vi "Hokuyo publish to ROS.vi"() -> ()   [LabVIEW 2014]
uses:
  Labview-ROS-Examples/Common/LaserScan.ctl
  <userlib>/ROS for LabVIEW Software/ROS/Code/Console/Servers/ServerSubs/TopicDef.ctl
  <userlib>/ROS for LabVIEW Software/ROS/Code/SubVIs/_ROSDirection.ctl
  <userlib>/ROS for LabVIEW Software/ROS/Code/_ROSDefinition.vi
  <instrlib>/Hokuyo URG Series/Public/Initialize-Standard.vi
  <instrlib>/Hokuyo URG Series/Hokuyo URG Series.lvlib
panel:
  out "LaserScan":T1
  out "end":bool
  in  "polar attributes (hidden)":T2={"maximum"=30000.0, "minimum"=0.0, "clip to min"=FALSE, "log?(F)"=TRUE, "grid color"=6710886, "plot color"=65280, "fmt and prec"={"format"=enum."Decimal", "precision"=0}, "visible section"=8} {"minimum" format="%0.2f"; "maximum" format="%0.2f"}
  in  "Protocol":u32(ring)=2 items=["Convert to Latest", "SCIP 1.1", "SCIP 2.0"]
  in  "ID Query?":bool=TRUE
  in  "Checksum":bool
  in  "VISA resource name":refnum<visa-resource-name>
  in  "Stop":bool
  out "Data Aquired":picture
  in  "Grid Color":u32(colorbox)=16777222
  in  "Plot Color":u32(colorbox)=6618880
  in  "Max (m)":dbl=4.1
  in  "End Point":dbl=120.0
  in  "Start Point":dbl=-120.0
  in  "Cluster Count":dbl=1.0
  in  "Encoding Width":u16(ring)=3 items=["2 Byte"=2, "3 Byte"=3]
  in  "ROS Master":string="172.16.0.10:11311"
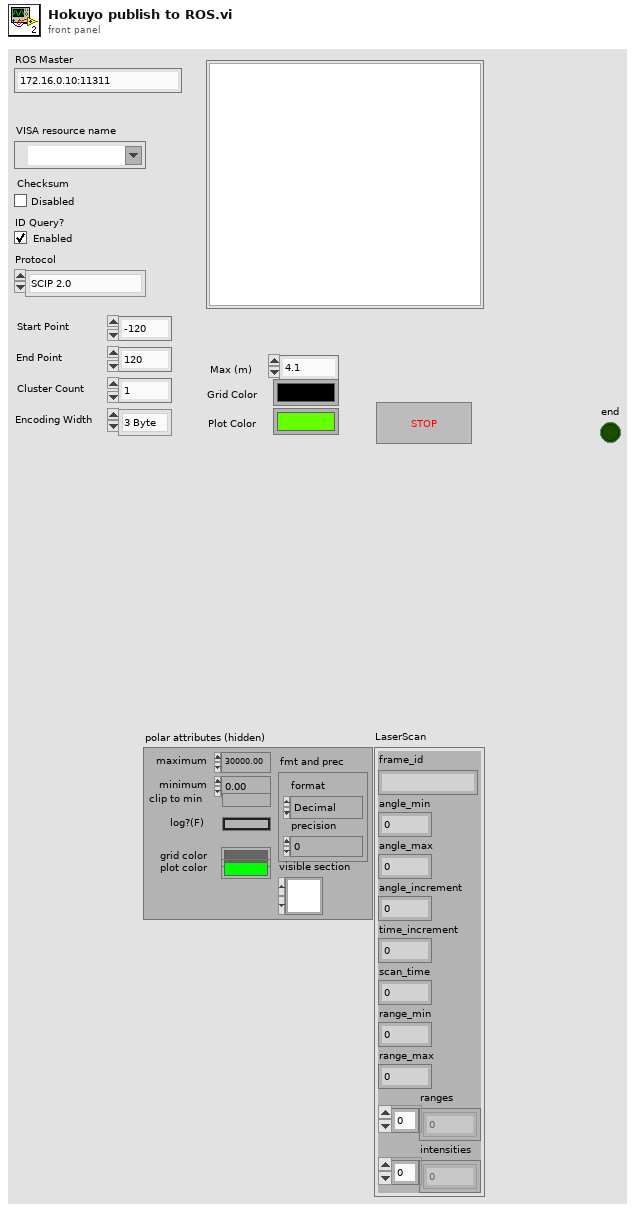
[diagram p1: front panel]
types:
  T1 = typedef "LaserScan.ctl" = cluster{"frame_id":string, "angle_min":dbl, "angle_max":dbl, "angle_increment":dbl, "time_increment":dbl, "scan_time":dbl, "range_min":dbl, "range_max":dbl, "ranges":dbl[], "intensities":dbl[]}
  T2 = cluster{"maximum":dbl, "minimum":dbl, "clip to min":bool, "log?(F)":bool, "grid color":u32, "plot color":u32, "fmt and prec":cluster{"format":enum8{"Decimal", "Scientific", "Engineering", "Binary", "Octal", "Hex"}, "precision":u8}, "visible section":u16}
  T3 = typedef "TopicDef.ctl" = cluster{"Topic":string, "Type":string, "Action":T4, "Update (ms)":u16, "queue size":u16}
  T4 = typedef "_ROSDirection.ctl" = enum16{"Node", "Publisher", "Subscriber", "ServiceClient", "ServiceProvider"}
  T5 = typedef "_ROSControl.ctl" = cluster{"topic port":u16, "Node":string, "topic":string, "type":string, "node port":u16, "error ":errorcluster, "Direction":T4, "Update (ms)":u16, "FIFO size":u16}
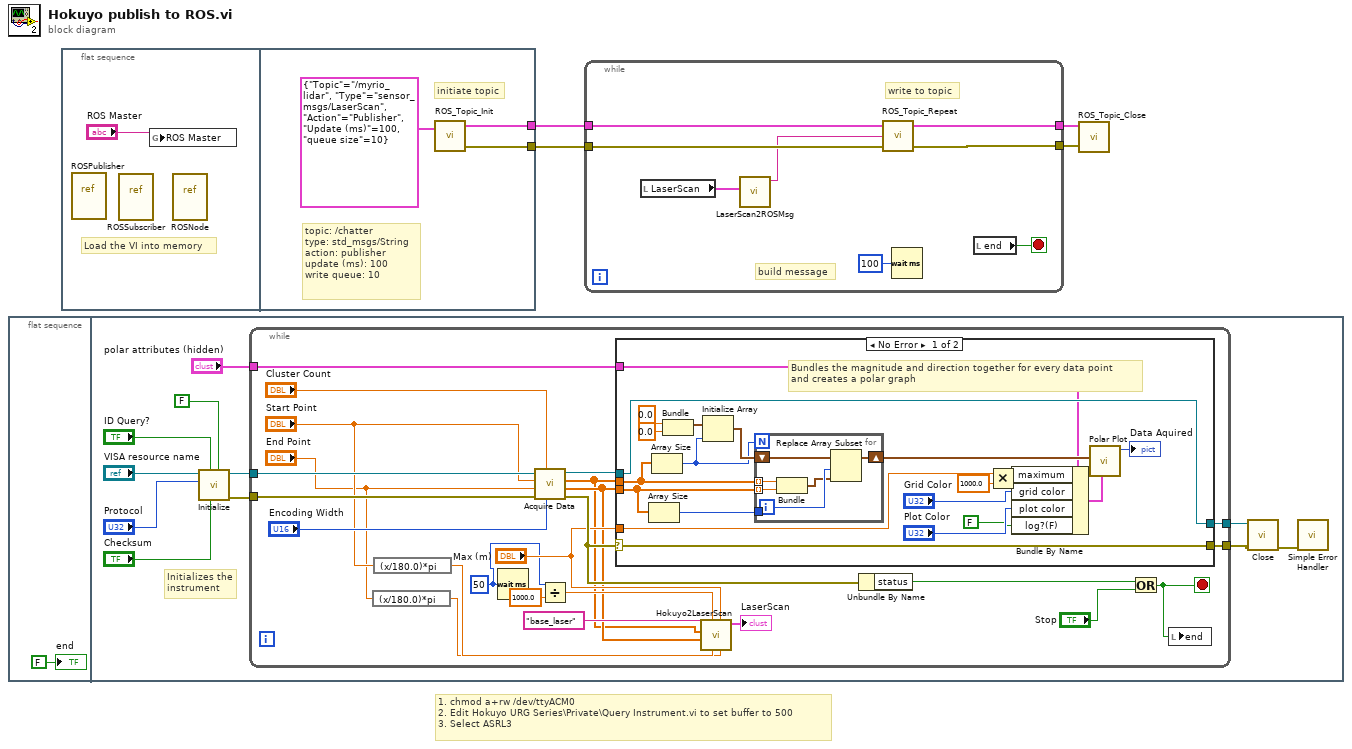
[diagram p0: block diagram]
diagram:
  # "1. chmod a+rw /dev/ttyACM0\n2. Edit Hokuyo URG Series\\Private\\Query Instrument.vi to set buffer to 500 \n3. Select ASRL3"
  n1 = flat-sequence {
    frame #0 {
      "end" <- FALSE ("end")
    }
    frame #1 {
      # "Initializes the instrument"
      n2 = call-poly <instrlib>:"Initialize.vi"("Reset? (F: No)"=FALSE ("Reset Instrument (Disabled)"), "Checksum (Disabled)"="Checksum", "ID Query? (Enabled)"="ID Query?", "Protocol (2: SCIP 2.0)"="Protocol", "VISA resource name"="VISA resource name") -> ("error out"=w7:errorcluster, "VISA resource name out"=w8:refnum<visa-resource-name>)  [unwired: 5 in]
      n3 = while {
        tunnel: w8 -> [w33]
        tunnel: [w40] -> w16
        tunnel: [w39] -> w9
        tunnel: w7 -> [w32]
        tunnel: "polar attributes (hidden)" -> [w31]
        stop <- w29 stop-if-true
        w19 = u32 50 ("milliseconds to wait")
        n4 = expression code="(x/180.0)*pi" ("degrees to radians")("End Point") -> (w24:dbl)
        n5 = expression code="(x/180.0)*pi" ("degrees to radians")("Start Point") -> (w26:dbl)
        n6 = Wait (ms)(milliseconds to wait=w19) -> ()  [unwired: 1 out]
        n7 = call <instrlib>:"Acquire Data.vi"("Data Encoding Width (3 Byte)"="Encoding Width", "Cluster Count (1)"="Cluster Count", "error in (no error)"=w32, "End Point (120°)"="End Point", "Start Point (-120°)"="Start Point", "VISA resource name"=w33) -> ("error out"=w35:errorcluster, "Direction"=w18:dbl[], "Magnitude"=w17:dbl[], "VISA resource name out"=w36:refnum<visa-resource-name>)  [unwired: 2 in]
        n8 = Divide(x=w19, y=1000.0) -> (x/y=w22:dbl)
        n9 = case shown="No Error" w35 {
          selector: w35 -> [w58 w68]
          tunnel: [w58 w68] -> w40
          tunnel: w36 -> [w59 w67]
          tunnel: [w59 w67] -> w39
          tunnel: w17 -> [w53 _]
          tunnel: w18 -> [w43 _]
          tunnel: w31 -> [w49 _]
          tunnel: "Max (m)" -> [w41 _]
          frame No Error {
            # "Bundles the magnitude and direction together for every data point\nand creates a polar graph"
            n10 = Array Size(array=w43) -> (size(s)=w42:i32)
            n11 = Array Size(array=w53) -> (size(s)=w52:i32)
            n12 = Bundle(0.0, 0.0) -> (w55:cluster{dbl, dbl})  [unwired: 1 in]
            n13 = Initialize Array(w55, w52) -> (w54:cluster{dbl, dbl}[])
            n14 = for {
              N: w52 -> [_]
              shift-right: [w62] -> w51
              shift-left: w54 -> [w63]
              tunnel: w53 -> [w66] mode=indexing
              tunnel: w43 -> [w65] mode=indexing
              tunnel: w42 -> [_]
              i -> [w64]
              n15 = Bundle(w66, w65) -> (w61:cluster{dbl, dbl})  [unwired: 1 in]
              n16 = Replace Array Subset(array=w63, new element=w61, index=w64) -> (w62:cluster{dbl, dbl}[])
            }
            n17 = Multiply(x=w41, y=1000.0) -> (x*y=w45:dbl)
            n18 = Bundle By Name(cluster=w49, "maximum"=w45, "grid color"="Grid Color", "plot color"="Plot Color", "log?(F)"=FALSE) -> (w50:T2)
            n19 = call <vilib>:"Polar Plot.vi"("polar attributes"=w50, "data array [mag, phase (deg)]"=w51) -> ("new picture"=→"Data Aquired":picture)  [unwired: 9 in]
          }
          frame Error {
          }
        }
        n20 = call "Hokuyo2LaserScan.vi"("angle_max"=w24, "range_max"="Max (m)", "angle_min"=w26, "scan_time"=w22, "Direction"=w18, "Magnitude"=w17, "frame_id"="base_laser") -> ("LaserScan"=→"LaserScan":T1)  [unwired: 4 in]
        n21 = Unbundle By Name(w35) -> ("status"=w38:bool)
        n22 = Or(x=w38, y="Stop") -> (x .or. y?=w29:bool)
        n23 = local write "end"(w29) -> ()
      }
      n24 = call <instrlib>:"Close.vi"("error in (no error)"=w16, "VISA resource name"=w9) -> ("error out"=w13:errorcluster)  [unwired: 9 in]
      n25 = call <vilib>:"Simple Error Handler.vi"("error in (no error)"=w13) -> ()  [unwired: 4 in, 5 out]
    }
  }
  n26 = flat-sequence {
    tunnel: [w71] -> w4
    tunnel: [w70] -> w3
    frame #0 {
      # "Load the VI into memory"
      n27 = vi-ref <userlib>:"ROSPublisher.vi"() -> ()  [unwired: 1 out]
      n28 = vi-ref <userlib>:"ROSSubscriber.vi"() -> ()  [unwired: 1 out]
      n29 = global write "_ROSDefinition.vi" "ROS Master"("ROS Master") -> ()
      n30 = vi-ref <userlib>:"ROSNode.vi"() -> ()  [unwired: 1 out]
    }
    frame #1 {
      # "topic: /chatter\ntype: std_msgs/String\naction: publisher\nupdate (ms): 100\nwrite queue: 10"
      # "initiate topic"
      n31 = call <userlib>:"ROS_Topic_Init.vi"("Definitions"=T3 {"Topic"="/myrio_lidar", "Type"="sensor_msgs/LaserScan", "Action"=enum."Publisher", "Update (ms)"=100, "queue size"=10}) -> ("ROS out"=w71:T5, "error out"=w70:errorcluster)  [unwired: 2 in]
    }
  }
  n32 = while {
    tunnel: w4 -> [w80]
    tunnel: w3 -> [w79]
    tunnel: [w78] -> w2
    tunnel: [w77] -> w1
    stop <- w76 stop-if-true
    # "build message"
    # "write to topic"
    n33 = local read "LaserScan"() -> (w75:T1)
    n34 = call "LaserScan2ROSMsg.vi"("LaserScan"=w75) -> ("msg out"=w74:string)  [unwired: 10 in]
    n35 = call <userlib>:"ROS_Topic_Repeat.vi"("error in (no error)"=w79, "Msg in"=w74, "ROS in"=w80) -> ("error out"=w77:errorcluster, "ROS out"=w78:T5)  [unwired: 1 in]
    n36 = Wait (ms)(milliseconds to wait=u32 100) -> ()  [unwired: 1 out]
    n37 = local read "end"() -> (w76:bool)
  }
  n38 = call <userlib>:"ROS_Topic_Close.vi"("error in"=w1, "ROS in"=w2) -> ()  [unwired: 2 in, 1 out]
